vi "Mcp2210 xfer Spi Data.vi"(0 "handle":i32, 1 "length":i32, 5 "Tx Data":u8[](array[numeric]) format="%02x", 7 "CS select one time":bool, 9 "pbaudRate":u32, 11 "error in (no error)":errorcluster, 12 "CS Pin Select":u32(ring) items=["CS0", "CS1", "CS2", "CS3", "CS4", "CS5", "CS6", "CS7", "CS8", "Use Default Setting"]) -> (4 "handle out":i32, 6 "RX Data":u8[](array[numeric]) format="%02x", 10 "pbaudRate out":u32, 15 "error out":errorcluster)   [LabVIEW 2015, in "mcp2210.lvlib"]
doc: "Data transfer over SPI bus. This API assumes that GPIO configuration and SPI\ncommunication settings are already configured, either as power-up default settings or through the use\nof Mcp2210_SetGpioConfig() and Mcp2210_SetSPIConfig(). In addition, this API offers the user the\noption to change the current (VM) SPI transfer length and/or to indicate which GPIO pin(s) to be used\nas CS pin(s). Please note that these changes are not reverted at the end of the SPI data transfer but\nremain in effect until a new GPIO/SPI configuration change is initiated by the user.\nIf SPI configuration change is not accepted (because SPI transfer is in progress) the API returns\nE_ERR_SPI_CFG_ABORT error.\nIn the case of the current (VM) SPI configuration change, the API call returns the actual configuration\nvalues that will be used by the device, derived from the user supplied ones but adapted to the\ndevice capabilities.\nThis API can also reverse the effect of the GP8 firmware error: when GP8 is set as GPIO \"out\",\nthe SPI transfer command is changing it to GPIO \"in\". The user has the option to skip this fix if the\napplication execution speed gain is relevant.\nParameters:\nInputs:\n- void *handle - The pointer to the device handle. Cannot be NULL.\n- unsigned char *pdataTx - data buffer to be transmitted. Cannot be NULL.\nThe user must ensure that buffer size matches the SPI transfer\nsize setting.\n- unsigned int *pbaudRate - SPI transfer speed. Cannot be NULL.\n- If the value is different than the current speed,\nthe API attempts to change it as requested.\n- If the value is 0, the current SPI transfer speed is preserved.\n- unsigned int *ptxferSize - Bytes to transfer per SPI transaction.\n- 16-bit value => max valid value is (2^16)-1.\n- A larger values than (2^16)-1 indicates that\nthe current SPI transfer size setting must remain unchanged.\n- If set to 0, all the configuration changes are accepted if\nvalid (baudRate, CS/GPIO configuration, transfer size set 0),\nbut no SPI transfer is performed.\n- Cannot be NULL.\n- unsigned int csmask - bit mask indicating which GPIO pins must be active chip select\n(CS) pins for the SPI transfer. It is assumed that CS settings\n(idle/active values and delays) are properly configured\nalready either as power-up defaults or with prior use\nof the Mcp2210_SetSPIConfig() API.\nbit31 - ... - - bit8 bit0\nGP8CE x ... x x CS8 CS7 CS6 CS5 CS4 CS3 CS2 CS1 CS0\n- A bit value of '1' configures the GPIO pins as CS\n(alternate function 1) during the SPI data transfer.\nA bit value of 0 configures the pins as GPIO (standard\nfunction) except the pins which are configuration as\ndedicated function (alternate function 2).\nThe GP direction and default values must be already configured\nas needed either as power-up defaults or with prior use of\nMcp2210_SetGpioConfig().\n- If all CS[0..8] bit values are '0', current GPIO configuration\nis preserved.\n- If csmask[31] bit (GP8CE) is set ('1'), the GP8 errata is\nignored, assuming that user application is not affected by the\nGP8 pin being reconfigured as GPIO \"input\" after the SPI\ntransfer command.\nOutputs:\n- unsigned char *pdataRx - receive data buffer. Cannot be NULL.\nThe user must ensure that buffer size matches the SPI transfer\nsize setting.\n- unsigned int *pbaudRate - If the function call returns E_SUCCESS, this parameter contains\nthe current transfer speed value accepted by the device.\nThe value may differ from the user supplied one - it may be\nderived from the user supplied value but adapted to the device\ncapabilities.\n- unsigned int *ptxferSize - If the function call returns E_SUCCESS, this parameter contains\nthe current transfer size used by the device.\nReturns:\n- 0 for success: E_SUCCESS\n- negative error code: E_ERR_NULL, E_ERR_INVALID_HANDLE_VALUE\nE_ERR_HID_TIMEOUT, E_ERR_HID_RW_FILEIO\nE_ERR_UNKOWN_ERROR, E_ERR_CMD_ECHO, E_ERR_CMD_FAILED\nE_ERR_SPI_TIMEOUT, E_ERR_SPI_EXTERN_MASTER, E_ERR_SPI_RX_INCOMPLETE\nE_ERR_SPI_CFG_ABORT\n\nMCP2210_DLL_UM_API int __stdcall Mcp2210_xferSpiData(void *handle, unsigned char *pdataTx, unsigned char *pdataRx,\n unsigned int *pbaudRate, unsigned int *ptxferSize, unsigned int csmask);"
uses:
  <userlib>/mcp2210/mcp2210.lvlib
  <userlib>/mcp2210/mcp2210_dll_um_x86.dll
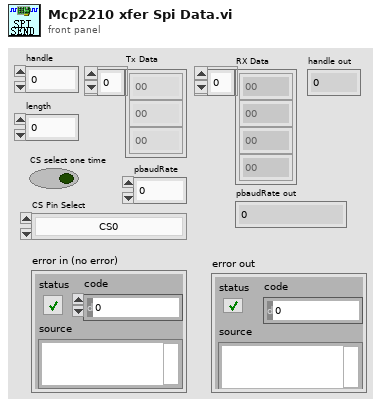
[diagram p1: front panel]
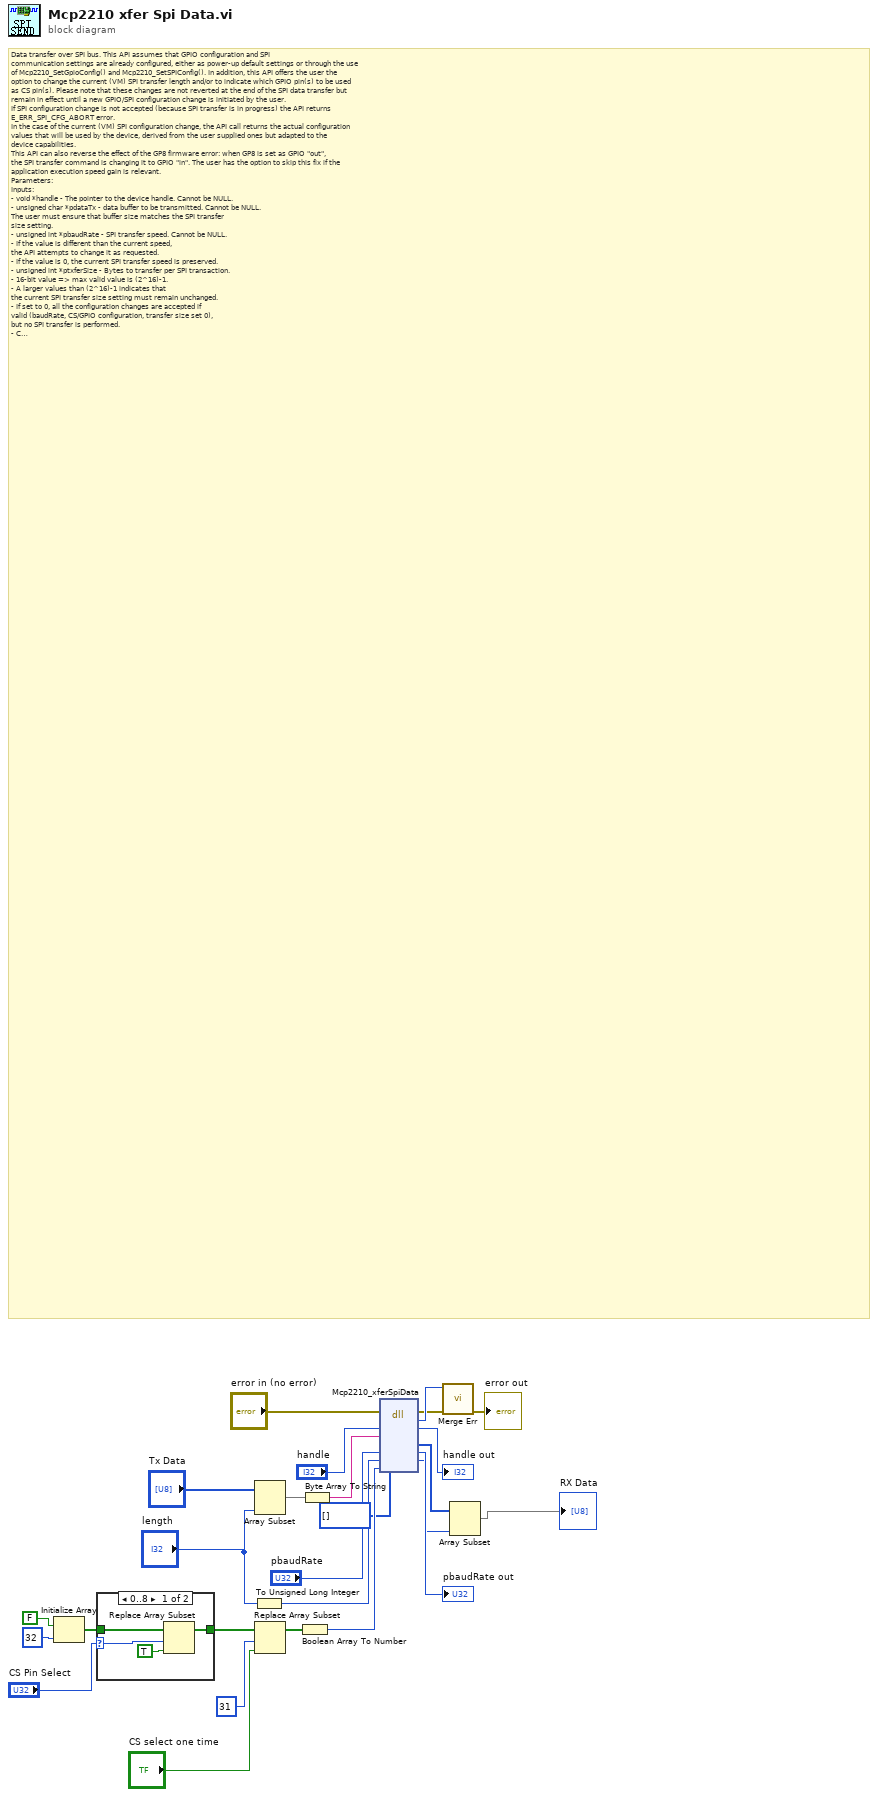
[diagram p0: block diagram]
diagram:
  # "Data transfer over SPI bus. This API assumes that GPIO configuration and SPI\ncommunication settings are already configured, either as power-up default settings or through the use\nof Mcp2210_SetGpioConfig() and Mcp2210_SetSPIConfig(). In addition, this API offers the user the\noption to change the current (VM) SPI transfer length and/or to indicate which GPIO pin(s) to be used\nas CS pin(s). Please note that these changes are not reverted at the end of the SPI data transfer but\nremain in effect until a new GPIO/SPI configuration change is initiated by the user.\nIf SPI configuration change is not accepted (because SPI transfer is in progress) the API returns\nE_ERR_SPI_CFG_ABORT error.\nIn the case of the current (VM) SPI configuration change, the API call returns the actual configuration\nvalues that will be used by the device, derived from the user supplied ones but adapted to the\ndevice capabilities.\nThis API can also reverse the effect of the GP8 firmware error: when GP8 is set as GPIO \"out\",\nthe SPI transfer command is changing it to GPIO \"in\". The user has the option to skip this fix if the\napplication execution speed gain is relevant.\nParameters:\nInputs:\n- void *handle - The pointer to the device handle. Cannot be NULL.\n- unsigned char *pdataTx - data buffer to be transmitted. Cannot be NULL.\nThe user must ensure that buffer size matches the SPI transfer\nsize setting.\n- unsigned int *pbaudRate - SPI transfer speed. Cannot be NULL.\n- If the value is different than the current speed,\nthe API attempts to change it as requested.\n- If the value is 0, the current SPI transfer speed is preserved.\n- unsigned int *ptxferSize - Bytes to transfer per SPI transaction.\n- 16-bit value => max valid value is (2^16)-1.\n- A larger values than (2^16)-1 indicates that\nthe current SPI transfer size setting must remain unchanged.\n- If set to 0, all the configuration changes are accepted if\nvalid (baudRate, CS/GPIO configuration, transfer size set 0),\nbut no SPI transfer is performed.\n- Cannot be NULL.\n- unsigned int csmask - bit mask indicating which GPIO pins must be active chip select\n(CS) pins for the SPI transfer. It is assumed that CS settings\n(idle/active values and delays) are properly configured\nalready either as power-up defaults or with prior use\nof the Mcp2210_SetSPIConfig() API.\nbit31 - ... - - bit8 bit0\nGP8CE x ... x x CS8 CS7 CS6 CS5 CS4 CS3 CS2 CS1 CS0\n- A bit value of '1' configures the GPIO pins as CS\n(alternate function 1) during the SPI data transfer.\nA bit value of 0 configures the pins as GPIO (standard\nfunction) except the pins which are configuration as\ndedicated function (alternate function 2).\nThe GP direction and default values must be already configured\nas needed either as power-up defaults or with prior use of\nMcp2210_SetGpioConfig().\n- If all CS[0..8] bit values are '0', current GPIO configuration\nis preserved.\n- If csmask[31] bit (GP8CE) is set ('1'), the GP8 errata is\nignored, assuming that user application is not affected by the\nGP8 pin being reconfigured as GPIO \"input\" after the SPI\ntransfer command.\nOutputs:\n- unsigned char *pdataRx - receive data buffer. Cannot be NULL.\nThe user must ensure that buffer size matches the SPI transfer\nsize setting.\n- unsigned int *pbaudRate - If the function call returns E_SUCCESS, this parameter contains\nthe current transfer speed value accepted by the device.\nThe value may differ from the user supplied one - it may be\nderived from the user supplied value but adapted to the device\ncapabilities.\n- unsigned int *ptxferSize - If the function call returns E_SUCCESS, this parameter contains\nthe current transfer size used by the device.\nReturns:\n- 0 for success: E_SUCCESS\n- negative error code: E_ERR_NULL, E_ERR_INVALID_HANDLE_VALUE\nE_ERR_HID_TIMEOUT, E_ERR_HID_RW_FILEIO\nE_ERR_UNKOWN_ERROR, E_ERR_CMD_ECHO, E_ERR_CMD_FAILED\nE_ERR_SPI_TIMEOUT, E_ERR_SPI_EXTERN_MASTER, E_ERR_SPI_RX_INCOMPLETE\nE_ERR_SPI_CFG_ABORT\n\nMCP2210_DLL_UM_API int __stdcall Mcp2210_xferSpiData(void *handle, unsigned char *pdataTx, unsigned char *pdataRx,\n                                                     unsigned int *pbaudRate, unsigned int *ptxferSize, unsigned int csmask);"
  n1 = Initialize Array(FALSE, 32 ("dimension size")) -> (w11:bool[])
  n2 = case shown="0..8" "CS Pin Select" {
    selector: "CS Pin Select" -> [w29 _]
    tunnel: w11 -> [w30 w31]
    tunnel: [w27 w31] -> w9
    frame 0..8 {
      n3 = Replace Array Subset(array=w30, new element=TRUE ("new element/subarray"), index=w29) -> (w27:bool[])
    }
    frame 9, Default {
    }
  }
  n4 = To Unsigned Long Integer(number="length") -> (unsigned 32bit integer=w19:u32)
  n5 = Array Subset(array="Tx Data", length="length") -> (w22:u8[])  [unwired: 1 in]
  n6 = Replace Array Subset(array=w9, new element="CS select one time", index=31) -> (w6:bool[])
  n7 = Boolean Array To Number(Boolean array=w6) -> (number=w7:u32)
  n8 = Byte Array To String(unsigned byte array=w22) -> (string=w21:string)
  n9 = dll-call lib="D:/LabVIEW 2015/user.lib/mcp2210/mcp2210_dll_um_x86.*" fn="Mcp2210_xferSpiData"(error in="error in (no error)", "handle"="handle", "pdataTx"=w21, "pdataRx"=u8[] [], "pbaudRate"="pbaudRate", "ptxferSize"=w19, "csmask"=w7) -> (error out=w15:errorcluster, "return type"=w17:i32, "handle"=→"handle out":i32, "pdataRx"=w3:u8[], "pbaudRate"=→"pbaudRate out":u32, "ptxferSize"=w2:u32)  [unwired: 4 in, 1 out]
  n10 = call <userlib>:"Merge Err.vi"("error in (no error)"=w15, "return type"=w17) -> ("error out"=→"error out":errorcluster)  [unwired: 9 in]
  n11 = Array Subset(array=w3, length=w2) -> (→"RX Data":u8[])  [unwired: 1 in]
